vi "ic_tester_panel.vi"() -> ()   [LabVIEW 2026]
panel:
  in  "Serial Port":refnum<visa-resource-name>="N/A"
  in  "stop":bool
  in  "Tab Control":enum32{"Integrated Circuit Testing"}(tab)
  out "Current":dbl(graph)
  in  "IC Select":u16(ring) items=["7408", "7432", "7404"]
  out "D1":bool
  out "D2":bool
  out "D3":bool
  out "D4":bool
  out "D5":bool
  out "D6":bool
  out "D8":bool
  out "D9":bool
  out "D10":bool
  out "D11":bool
  out "D12":bool
  out "D13":bool
  in  "Start Test":bool
  out "Tests Ran":dbl
  out "PASS":bool
  out "FAIL":bool
  out "Passed":dbl
  out "Failed":dbl
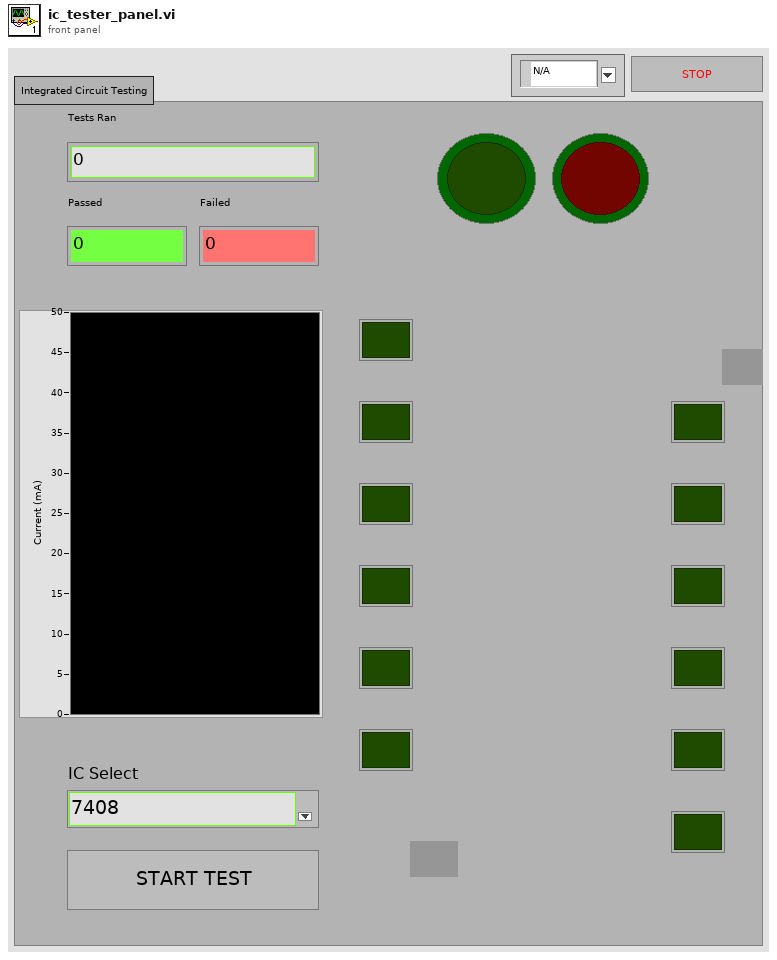
[diagram p1: front panel]
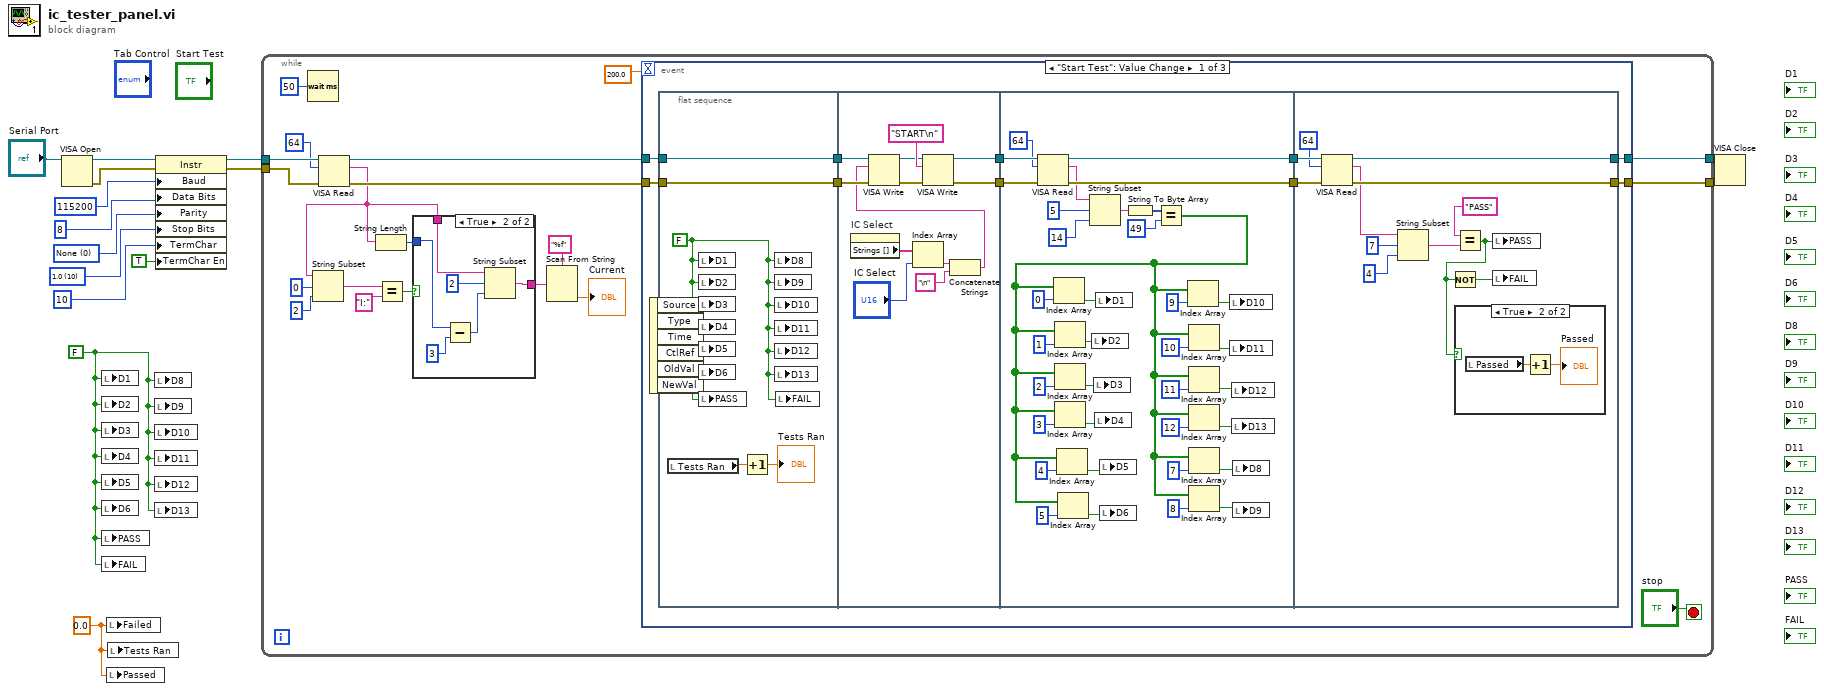
[diagram p0: block diagram]
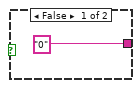
[diagram p2: hidden frame]
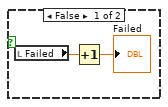
[diagram p3: hidden frame]
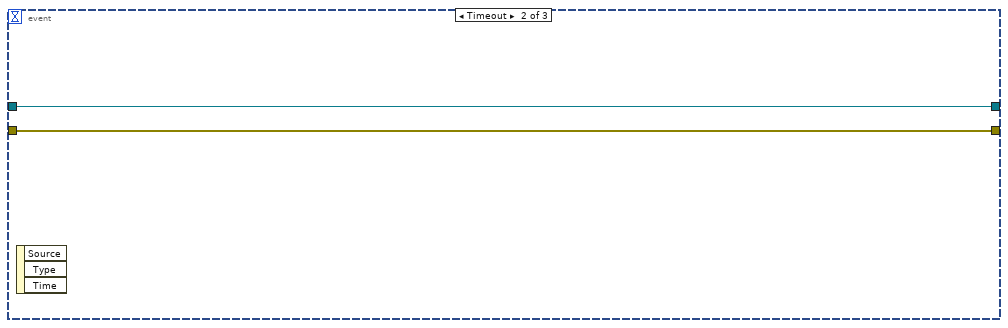
[diagram p4: hidden frame]
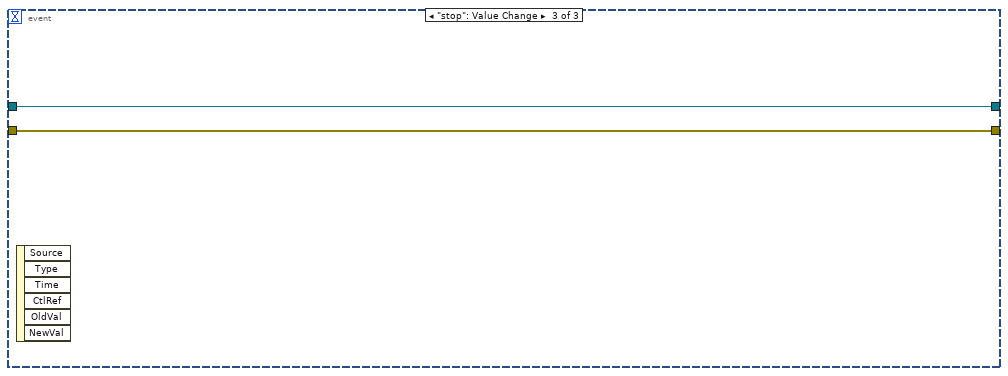
[diagram p5: hidden frame]
diagram:
  w1 = 0.0 ("Failed")
  w2 = FALSE ("D1")
  w7 = u16 10 items=["1.0"=10, "1.5"=15, "2.0"=20] ("Serial Settings:Stop Bits")
  w8 = u16 0 items=["None", "Odd", "Even", "Mark", "Space"] ("Serial Settings:Parity")
  n1 = VISA Open(VISA resource name="Serial Port") -> (VISA resource name=w14:refnum<visa-resource-name>, error out=w12:errorcluster)  [unwired: 4 in]
  n2 = local write "D1"(w2) -> ()
  n3 = local write "D2"(w2) -> ()
  n4 = local write "D3"(w2) -> ()
  n5 = local write "D4"(w2) -> ()
  n6 = local write "D5"(w2) -> ()
  n7 = local write "D6"(w2) -> ()
  n8 = local write "PASS"(w2) -> ()
  n9 = local write "FAIL"(w2) -> ()
  n10 = local write "Failed"(w1) -> ()
  n11 = local write "Passed"(w1) -> ()
  n12 = local write "Tests Ran"(w1) -> ()
  n13 = local write "D8"(w2) -> ()
  n14 = local write "D9"(w2) -> ()
  n15 = local write "D10"(w2) -> ()
  n16 = local write "D11"(w2) -> ()
  n17 = local write "D12"(w2) -> ()
  n18 = local write "D13"(w2) -> ()
  n19 = property class="Instr"(reference=w14, error in=w12, "Baud"=u32 115200 ("Serial Settings:Baud Rate"), "Data Bits"=u16 8 ("Serial Settings:Data Bits"), "Parity"=w8, "Stop Bits"=w7, "TermChar"=u8 10 ("Message Based Settings:Termination Character"), "TermChar En"=TRUE ("Message Based Settings:Termination Character Enable")) -> (reference out=w13:refnum<visa-resource-name>, error out=w11:errorcluster)
  n20 = while {
    tunnel: w13 -> [w34]
    tunnel: w11 -> [w32]
    tunnel: [w29] -> w4
    tunnel: [w28] -> w3
    stop <- "stop" stop-if-true
    n21 = Wait (ms)(milliseconds to wait=u32 50) -> ()  [unwired: 1 out]
    n22 = VISA Read(VISA resource name=w34, byte count=u32 64, error in (no error)=w32) -> (VISA resource name out=w31:refnum<visa-resource-name>, read buffer=w22:string, error out=w30:errorcluster)  [unwired: 1 out]
    n23 = String Subset(string=w22, offset (0)=0, length (rest)=2 ("length (rest)")) -> (substring=w21:string)
    n24 = String Length(string=w22) -> (length=w23:i32)
    n25 = Equal?(x=w21, y="I:") -> (x = y?=w20:bool)
    n26 = case shown="True" w20 {
      tunnel: w23 -> [_ w41]
      tunnel: ["0" w38] -> w18
      tunnel: w22 -> [_ w37]
      frame False {
      }
      frame True {
        n27 = Subtract(x=w41, y=3) -> (x-y=w39:i32)
        n28 = String Subset(string=w37, offset (0)=2, length (rest)=w39) -> (substring=w38:string)
      }
    }
    n29 = Scan From String(format string="%f", input string=w18) -> (output 1=→"Current":dbl)  [unwired: 3 in, 3 out]
    n30 = event shown="[0] \"Start Test\": Value Change" {
      selector: _ -> [_ _ _]
      dyn-events: _ -> [_ _ _]
      timeout: 200.0 -> [_ _ _]
      tunnel: w31 -> [w51 w123 w125]
      tunnel: w30 -> [w49 w122 w124]
      tunnel: [w48 w123 w125] -> w29
      tunnel: [w47 w122 w124] -> w28
      event "Start Test": Value Change {
        n31 = event-data() -> ()  [unwired: 1 in, 6 out]
        n32 = flat-sequence {
          tunnel: [w57] -> w52
          tunnel: w51 -> [w57]
          tunnel: [w56] -> w50
          tunnel: w49 -> [w56]
          tunnel: w52 -> [w66]
          tunnel: w50 -> [w64]
          tunnel: [w69] -> w46
          tunnel: [w68] -> w45
          tunnel: w46 -> [w104]
          tunnel: w45 -> [w105]
          tunnel: [w103] -> w44
          tunnel: [w102] -> w43
          tunnel: [w114] -> w47
          tunnel: [w115] -> w48
          tunnel: w44 -> [w117]
          tunnel: w43 -> [w116]
          frame #0 {
            w55 = FALSE ("D1")
            n33 = local read "Tests Ran"() -> (w54:dbl)
            n34 = local write "D1"(w55) -> ()
            n35 = local write "D2"(w55) -> ()
            n36 = local write "D3"(w55) -> ()
            n37 = local write "D4"(w55) -> ()
            n38 = local write "D5"(w55) -> ()
            n39 = local write "D6"(w55) -> ()
            n40 = local write "PASS"(w55) -> ()
            n41 = Increment(x=w54) -> (x+1=→"Tests Ran":dbl)
            n42 = local write "D8"(w55) -> ()
            n43 = local write "D9"(w55) -> ()
            n44 = local write "D10"(w55) -> ()
            n45 = local write "D11"(w55) -> ()
            n46 = local write "D12"(w55) -> ()
            n47 = local write "D13"(w55) -> ()
            n48 = local write "FAIL"(w55) -> ()
          }
          frame #1 {
            n49 = property on="IC Select" class="Ring (strict)"() -> ("Strings []"=w62:string[])  [unwired: 2 in, 2 out]
            n50 = Index Array(array=w62, index="IC Select") -> (element=w60:string)
            n51 = Concatenate Strings(w60, "\n" ("string")) -> (w58:string)
            n52 = VISA Write(VISA resource name=w66, write buffer=w58, error in (no error)=w64) -> (VISA resource name out=w65:refnum<visa-resource-name>, error out=w63:errorcluster)  [unwired: 1 out]
            n53 = VISA Write(VISA resource name=w65, write buffer="START\n", error in (no error)=w63) -> (VISA resource name out=w69:refnum<visa-resource-name>, error out=w68:errorcluster)  [unwired: 1 out]
          }
          frame #2 {
            n54 = VISA Read(VISA resource name=w104, byte count=u32 64, error in (no error)=w105) -> (VISA resource name out=w103:refnum<visa-resource-name>, read buffer=w96:string, error out=w102:errorcluster)  [unwired: 1 out]
            n55 = String Subset(string=w96, offset (0)=5, length (rest)=14 ("length (rest)")) -> (substring=w100:string)
            n56 = String To Byte Array(string=w100) -> (unsigned byte array=w99:u8[])
            n57 = Equal?(x=w99, y=u8 49) -> (x = y?=w71:bool[])
            n58 = Index Array(array=w71, index=0) -> (element=w95:bool)
            n59 = Index Array(array=w71, index=1) -> (element=w91:bool)
            n60 = Index Array(array=w71, index=2) -> (element=w90:bool)
            n61 = Index Array(array=w71, index=3) -> (element=w93:bool)
            n62 = Index Array(array=w71, index=4) -> (element=w94:bool)
            n63 = Index Array(array=w71, index=5) -> (element=w92:bool)
            n64 = local write "D2"(w91) -> ()
            n65 = local write "D3"(w90) -> ()
            n66 = local write "D4"(w93) -> ()
            n67 = local write "D1"(w95) -> ()
            n68 = local write "D5"(w94) -> ()
            n69 = local write "D6"(w92) -> ()
            n70 = Index Array(array=w71, index=9) -> (element=w81:bool)
            n71 = Index Array(array=w71, index=10) -> (element=w80:bool)
            n72 = Index Array(array=w71, index=11) -> (element=w79:bool)
            n73 = Index Array(array=w71, index=12) -> (element=w78:bool)
            n74 = Index Array(array=w71, index=7) -> (element=w83:bool)
            n75 = Index Array(array=w71, index=8) -> (element=w82:bool)
            n76 = local write "D10"(w81) -> ()
            n77 = local write "D11"(w80) -> ()
            n78 = local write "D12"(w79) -> ()
            n79 = local write "D13"(w78) -> ()
            n80 = local write "D8"(w83) -> ()
            n81 = local write "D9"(w82) -> ()
          }
          frame #3 {
            n82 = VISA Read(VISA resource name=w117, byte count=u32 64, error in (no error)=w116) -> (VISA resource name out=w115:refnum<visa-resource-name>, read buffer=w110:string, error out=w114:errorcluster)  [unwired: 1 out]
            n83 = String Subset(string=w110, offset (0)=7, length (rest)=4 ("length (rest)")) -> (substring=w106:string)
            n84 = Equal?(x="PASS", y=w106) -> (x = y?=w107:bool)
            n85 = Not(x=w107) -> (.not. x?=w109:bool)
            n86 = case shown="True" w107 {
              frame False {
                n87 = local read "Failed"() -> (w118:dbl)
                n88 = Increment(x=w118) -> (x+1=→"Failed":dbl)
              }
              frame True {
                n89 = local read "Passed"() -> (w120:dbl)
                n90 = Increment(x=w120) -> (x+1=→"Passed":dbl)
              }
            }
            n91 = local write "PASS"(w107) -> ()
            n92 = local write "FAIL"(w109) -> ()
          }
        }
      }
      event Timeout {
        n93 = event-data() -> ()  [unwired: 1 in, 3 out]
      }
      event "stop": Value Change {
        n94 = event-data() -> ()  [unwired: 1 in, 6 out]
      }
    }
  }
  n95 = VISA Close(VISA resource name=w4, error in (no error)=w3) -> ()  [unwired: 1 out]
